vi "texto.vi"() -> ()   [LabVIEW 2018]
uses:
  <vilib>/Analysis/Matrix/Datatypes/RealMatrix.ctl
  <vilib>/Utility/file.llb/Read Delimited Spreadsheet (DBL).vi
  <vilib>/Analysis/Matrix/Numeric/Conversions/Array To Matrix - RA2.vi
  <vilib>/Analysis/Matrix/Numeric/Conversions/Matrix To Array - RM.vi
  <vilib>/Utility/file.llb/Write Delimited Spreadsheet (DBL).vi
  <vilib>/Analysis/Matrix/NI_Matrix.lvlib
panel:
  in  "file (use dialog) 2":path
  out "Real Matrix":T1
  out "cluster":T2
  out "subarray":dbl[][](array[numeric])
  out "first row":dbl[](array[numeric])
  out "all rows":dbl[][](array[numeric])
  out "text":string
  in  "file (use dialog)":path
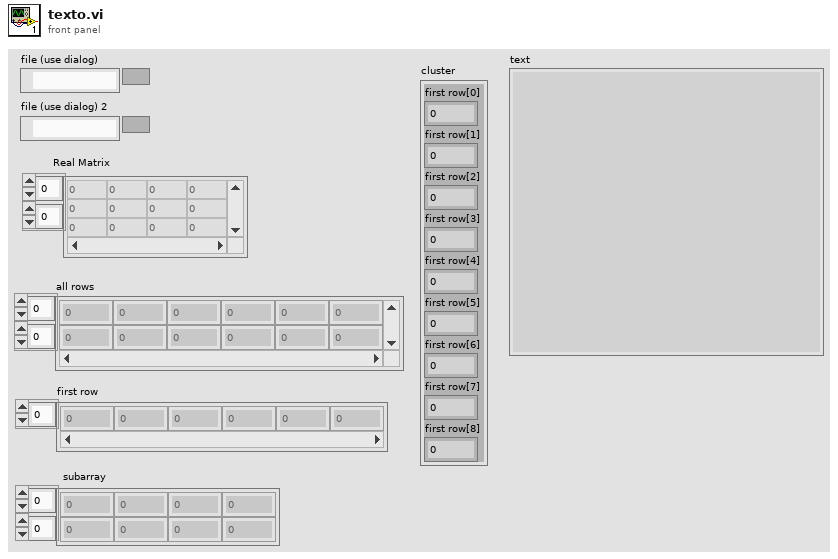
[diagram p1: front panel]
types:
  T1 = typedef "NI_Matrix.lvlib/RealMatrix.ctl" = dbl[][]
  T2 = cluster{"first row[0]":dbl, "first row[1]":dbl, "first row[2]":dbl, "first row[3]":dbl, "first row[4]":dbl, "first row[5]":dbl, "first row[6]":dbl, "first row[7]":dbl, "first row[8]":dbl}
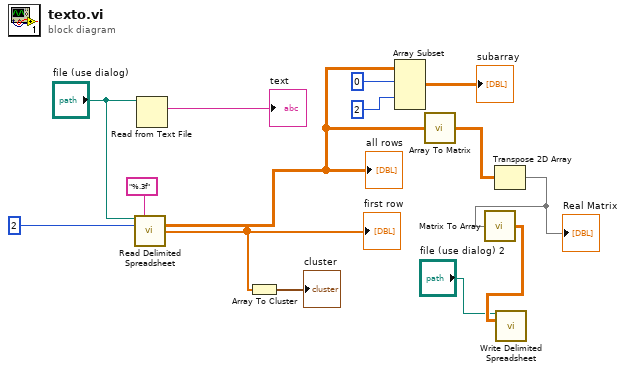
[diagram p0: block diagram]
diagram:
  n1 = call-poly <vilib>:"Read Delimited Spreadsheet.vi"("file path (dialog if empty)"="file (use dialog)", "format (%.3f)"="%.3f", "number of rows (all:-1)"=2) -> ("all rows"=w5:dbl[][], "first row"=w7:dbl[])  [unwired: 7 in, 4 out]
  "all rows" <- w5
  "first row" <- w7
  n2 = Read from Text File(file (use dialog)="file (use dialog)") -> (text=→"text":string)  [unwired: 3 in, 3 out]
  n3 = Array To Cluster(array=w7) -> (cluster=→"cluster":T2)
  n4 = Array Subset(array=w5, index (row)=0, index (col)=2 ("index")) -> (→"subarray":dbl[][])  [unwired: 2 in]
  n5 = call-poly <vilib>:"Array To Matrix.vi"("Real 2D Array"=w5) -> ("Real Matrix"=w4:T1)
  n6 = Transpose 2D Array(2D array=w4) -> (transposed array=w3:T1)
  "Real Matrix" <- w3
  n7 = call-poly <vilib>:"Matrix To Array.vi"("Real Matrix"=w3) -> ("Real 2D Array"=w2:dbl[][])
  n8 = call-poly <vilib>:"Write Delimited Spreadsheet.vi"("file path (dialog if empty)"="file (use dialog) 2", "2D data"=w2) -> ()  [unwired: 12 in, 2 out]
